vi "Populate Connection Source List.vi"(6 "initial Source":string, 8 "Alias Mappings by Module":T3[](array[typedef]), 9 "Possible Connections":T1[](array[typedef]), 10 "Module Index":i32, 11 "Source Reference":refnum<vi>) -> (2 "Endpoint List":string[](array[string]), 3 "Alias List":string[](array[string]))   [LabVIEW 2020, in "Routing and Faulting System Explorer.lvlib"]
uses:
  Routing and Faulting System Explorer.lvlib
  Alias Map by Module.ctl
  Possible Connections.ctl
  Shared/Routing and Faulting Hardware API/Types/Possible Connections for Endpoint.ctl
  Shared/Routing and Faulting Hardware API/Routing and Faulting Hardware API.lvlib
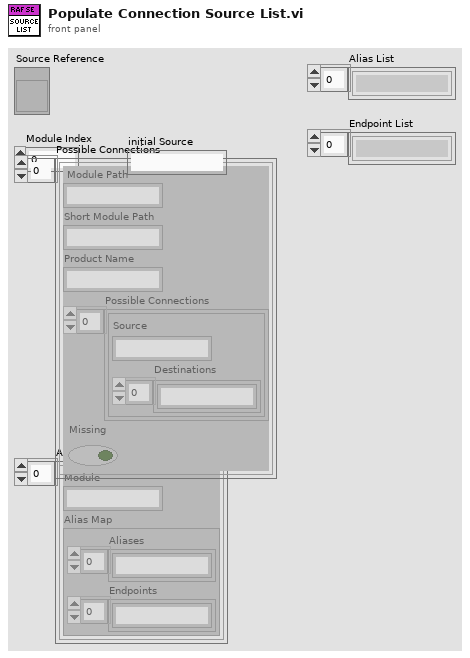
[diagram p1: front panel]
types:
  T1 = typedef "Routing and Faulting System Explorer.lvlib/Possible Connections.ctl" = cluster{" Module Path":string, "Short Module Path":string, "Product Name":string, "Possible Connections":T2[], "Missing":bool}
  T2 = typedef "Routing and Faulting Hardware API.lvlib/Possible Connections for Endpoint.ctl" = cluster{"Source":string, "Destinations":string[]}
  T3 = typedef "Routing and Faulting System Explorer.lvlib/Alias Map by Module.ctl" = cluster{"Module":string, "Alias Map":cluster{"Aliases":string[], "Endpoints":string[]}}
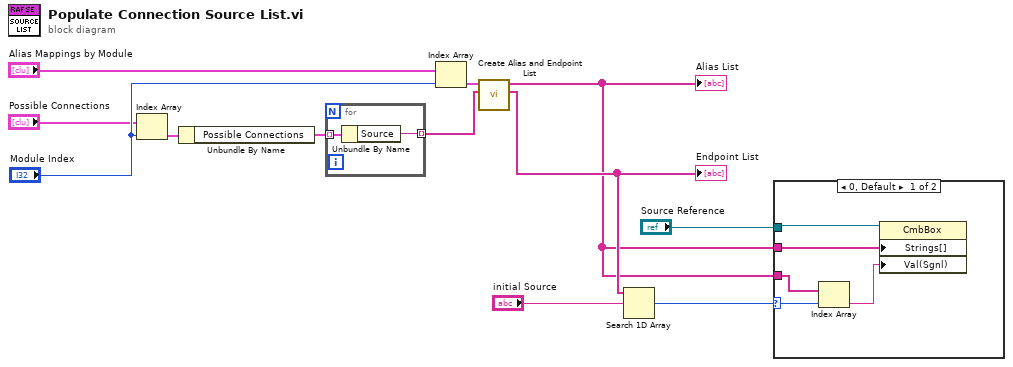
[diagram p0: block diagram]
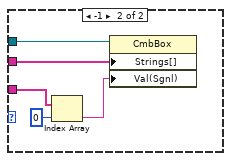
[diagram p2: hidden frame]
diagram:
  n1 = Index Array(array="Possible Connections", index="Module Index") -> (element=w7:T1)
  n2 = Unbundle By Name(w7) -> ("Possible Connections"=w6:T2[])
  n3 = for {
    tunnel: w6 -> [w14] mode=indexing
    tunnel: [w13] -> w11 mode=indexing
    n4 = Unbundle By Name(w14) -> ("Source"=w13:string)
  }
  n5 = Index Array(array="Alias Mappings by Module", index="Module Index") -> (element=w10:T3)
  n6 = call "Create Alias and Endpoint List.vi"("Endpoints"=w11, "Alias Mapping"=w10) -> ("Endpoint List"=w5:string[], "Alias List"=w1:string[])  [unwired: 8 in]
  "Endpoint List" <- w5
  "Alias List" <- w1
  n7 = Search 1D Array(1D array=w5, element="initial Source") -> (index of element=w3:i32)  [unwired: 1 in]
  n8 = case shown="0, Default" w3 {
    selector: w3 -> [w19 _]
    tunnel: w1 -> [w18 w24]
    tunnel: "Source Reference" -> [w15 w23]
    tunnel: w1 -> [w16 w22]
    frame 0, Default {
      n9 = Index Array(array=w18, index=w19) -> (element=w17:string)
      n10 = property on="Property Node" class="CmbBox"(reference=w15, "Strings[]"=w16, "Val(Sgnl)"=w17) -> ()  [unwired: 1 in, 2 out]
    }
    frame -1 {
      n11 = Index Array(array=w24, index=0) -> (element=w21:string)
      n12 = property on="Property Node" class="CmbBox"(reference=w23, "Strings[]"=w22, "Val(Sgnl)"=w21) -> ()  [unwired: 1 in, 2 out]
    }
  }
